vi "Emballage_BDD_GFS4470_CmdOn.vi"(8 "error in (no error)":errorcluster, 10 "TimeOut (sec)":dbl=3.0 format="%#_13g", 11 "VISA Datalogic 5":refnum<visa-resource-name>="COM7") -> (0 "sortie d'erreur":errorcluster, 1 "TIMEOUT_FIN?":bool, 2 "buffer de lecture":string, 3 "Nom de ressource VISA en sortie":refnum<visa-resource-name>)   [LabVIEW 2020]
panel:
  out "Barre graduée horizontale":u8(slide) scale=0.0..100.0
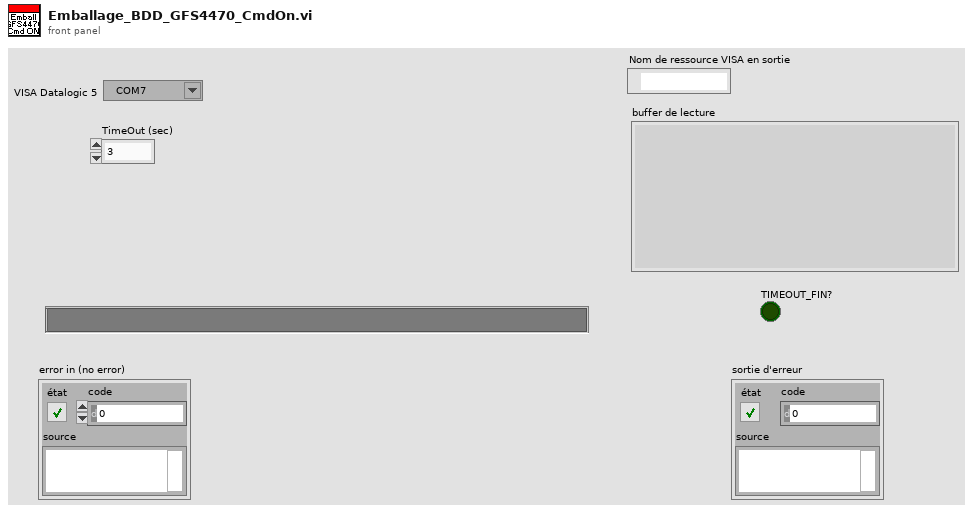
[diagram p1: front panel]
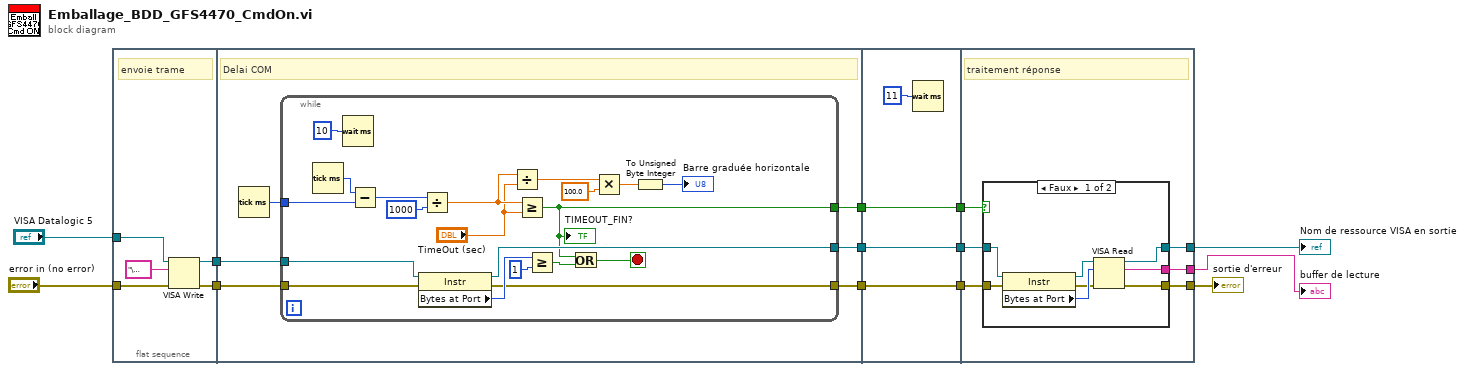
[diagram p0: block diagram]
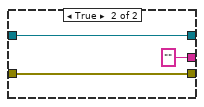
[diagram p2: hidden frame]
diagram:
  n1 = flat-sequence {
    tunnel: [w18] -> w9
    tunnel: [w17] -> w8
    tunnel: "VISA Datalogic 5" -> [w15]
    tunnel: "error in (no error)" -> [w14]
    tunnel: w9 -> [w21]
    tunnel: w8 -> [w23]
    tunnel: [w20] -> w7
    tunnel: [w22] -> w6
    tunnel: [w19] -> w5
    tunnel: w7 -> [w45]
    tunnel: w6 -> [w48]
    tunnel: [w45] -> w3
    tunnel: [w48] -> w4
    tunnel: w5 -> [w46]
    tunnel: [w46] -> w2
    tunnel: [w50] -> w11
    tunnel: w4 -> [w53]
    tunnel: w3 -> [w54]
    tunnel: w2 -> [w52]
    tunnel: [w51] -> w10
    tunnel: [w49] -> w1
    frame #0 {
      # "envoie trame"
      n2 = VISA Write(VISA resource name=w15, write buffer="\u0002", error in (no error)=w14) -> (VISA resource name out=w17:refnum<visa-resource-name>, error out=w18:errorcluster)  [unwired: 1 out]
    }
    frame #1 {
      # "Delai COM"
      n3 = Tick Count (ms)() -> (millisecond timer value=w24:u32)
      n4 = while {
        tunnel: w23 -> [w43]
        tunnel: w24 -> [w38]
        tunnel: [w28] -> w22
        tunnel: w21 -> [w27]
        tunnel: [w26] -> w20
        tunnel: [w25] -> w19
        stop <- w35 stop-if-true
        n5 = Tick Count (ms)() -> (millisecond timer value=w39:u32)
        n6 = Wait (ms)(milliseconds to wait=10 ("y")) -> ()  [unwired: 1 out]
        n7 = Subtract(x=w39, y=w38) -> (x-y=w37:u32)
        n8 = property class="Instr"(reference=w43, error in=w27) -> (reference out=w28:refnum<visa-resource-name>, error out=w26:errorcluster, "Bytes at Port"=w42:u32)
        n9 = Divide(x=w37, y=u32 1000) -> (x/y=w31:dbl)
        n10 = Divide(x=w31, y="TimeOut (sec)") -> (x/y=w34:dbl)
        n11 = Greater Or Equal?(x=w31, y="TimeOut (sec)") -> (x >= y?=w25:bool)
        "TIMEOUT_FIN?" <- w25
        n12 = Greater Or Equal?(x=w42, y=u32 1) -> (x >= y?=w40:bool)
        n13 = Or(x=w25, y=w40) -> (x .or. y?=w35:bool)
        n14 = Multiply(x=w34, y=100.0) -> (x*y=w33:dbl)
        n15 = To Unsigned Byte Integer(number=w33) -> (unsigned 8bit integer=→"Barre graduée horizontale":u8)
      }
    }
    frame #2 {
      n16 = Wait (ms)(milliseconds to wait=u32 11 ("attente (ms)")) -> ()  [unwired: 1 out]
    }
    frame #3 {
      # "traitement réponse"
      n17 = case shown="Faux" w52 {
        tunnel: [w61 w65] -> w50
        tunnel: w54 -> [w57 w65]
        tunnel: w53 -> [w56 w63]
        tunnel: [w62 "" ("message")] -> w51
        tunnel: [w55 w63] -> w49
        frame False {
          n18 = property class="Instr"(reference=w56, error in=w57) -> (reference out=w59:refnum<visa-resource-name>, error out=w58:errorcluster, "Bytes at Port"=w60:u32)
          n19 = VISA Read(VISA resource name=w59, byte count=w60, error in (no error)=w58) -> (VISA resource name out=w55:refnum<visa-resource-name>, read buffer=w62:string, error out=w61:errorcluster)  [unwired: 1 out]
        }
        frame True {
        }
      }
    }
  }
  "sortie d'erreur" <- w11
  "buffer de lecture" <- w10
  "Nom de ressource VISA en sortie" <- w1
